vi "ITC panel controller.vi"(6 "itc box state":T1={"ITC503 Address"="GPIB0::15::INSTR", "ITC temperature"=0.0, "ITC set temperature"=300.0, "heater"=300.0, "gas flow"=1.6, "P"=0.0, "D"=10.0, "I"=0.1, "ITC state"="X0A1C2S01H1L0\r", "nonzero temperature"=0.0, "Magn Field (T)"=0.0}, 7 "action":T4(ring), 8 "ITC panel IN":refnum<vi>, 11 "ITC panel IN":T5={"Locked"=FALSE, "Unlocked"=FALSE, "Remote"=FALSE, "Local"=FALSE, "in sweep"=FALSE, "start/stop sweep"=FALSE, "Sweep indicator"="X0A1C2S01H1L0\r", "heater MANUAL"=FALSE, "heater AUTO"=FALSE, "ITC state"="X0A1C2S01H1L0\r", "gas MANUAL"=FALSE, "gas AUTO"=FALSE, "heater"=13.5, "gas flow %"=0.0} {"gas flow %" format="%.3g"; "heater" format="%.3g"}) -> (3 "ITC panel OUT":T5={"Locked"=FALSE, "Unlocked"=FALSE, "Remote"=FALSE, "Local"=FALSE, "in sweep"=FALSE, "start/stop sweep"=FALSE, "Sweep indicator"="X0A1C2S01H1L0\r", "heater MANUAL"=FALSE, "heater AUTO"=FALSE, "ITC state"="X0A1C2S01H1L0\r", "gas MANUAL"=FALSE, "gas AUTO"=FALSE, "heater"=13.5, "gas flow %"=0.0} {"gas flow %" format="%.3g"; "heater" format="%.3g"})   [LabVIEW 2014]
uses:
  ITC Panel.ctl
  state.ctl
  Sample_Temperature_Source_Control.ctl
  itc 503 box state.ctl
  <vilib>/regexp/Match Regular Expression.xnode
panel:
  in  "temperature boxes":T2={"LTC21 Address"="GPIB0::15::INSTR", "ITC503 Address"="GPIB0::23::INSTR", "ITC temperature"=480.0, "ITC set temperature"=480.0, "LTC temperature"=0.0, "heater"=13.5, "gas flow"=0.0, "P"=10.0, "D"=1.0, "I"=3.0, "ITC state"="X0A1C2S01H1L0\r", "nonzero temperature"=0.0, "Magn Field (T)"=0.0, "LakeShore340"="", "LS340 Adress"=0, "Sample Temperature Source"=enum."read T <- LakeShore 340", "Neocera sensor"=1}
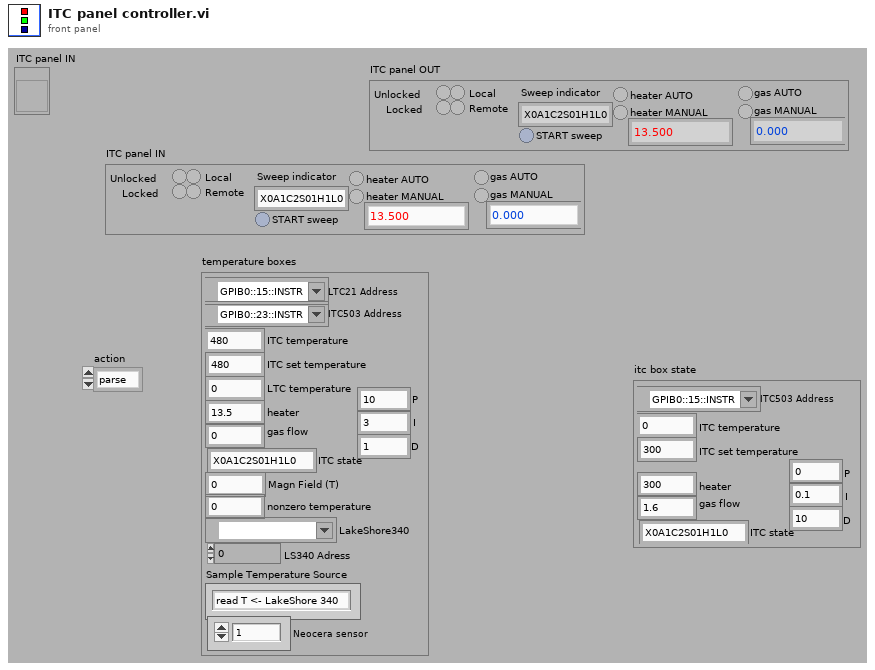
[diagram p1: front panel]
types:
  T1 = typedef "itc 503 box state.ctl" = cluster{"ITC503 Address":refnum<visa-resource-name>, "ITC temperature":dbl, "ITC set temperature":dbl, "heater":dbl, "gas flow":dbl, "P":dbl, "D":dbl, "I":dbl, "ITC state":string, "nonzero temperature":dbl, "Magn Field (T)":dbl}
  T2 = typedef "state.ctl" = cluster{"LTC21 Address":refnum<visa-resource-name>, "ITC503 Address":refnum<visa-resource-name>, "ITC temperature":dbl, "ITC set temperature":dbl, "LTC temperature":dbl, "heater":dbl, "gas flow":dbl, "P":dbl, "D":dbl, "I":dbl, "ITC state":string, "nonzero temperature":dbl, "Magn Field (T)":dbl, "LakeShore340":refnum<visa-resource-name>, "LS340 Adress":i16, "Sample Temperature Source":T3, "Neocera sensor":i32}
  T3 = typedef "Sample_Temperature_Source_Control.ctl" = enum16{"read T <- LakeShore 340", "read T <- Neocera"}
  T4 = enum16{"parse", "start sweep", "stop sweep", "heater auto", "heater manual", "set heater"}
  T5 = typedef "ITC Panel.ctl" = cluster{"Locked":bool, "Unlocked":bool, "Remote":bool, "Local":bool, "in sweep":bool, "start/stop sweep":bool, "Sweep indicator":string, "heater MANUAL":bool, "heater AUTO":bool, "ITC state":string, "gas MANUAL":bool, "gas AUTO":bool, "heater":dbl, "gas flow %":dbl}
  T6 = cluster{"Locked":bool, "Unlocked":bool, "Remote":bool, "Local":bool, "in sweep":bool, "start/stop sweep":bool, "Sweep indicator":string, "heater MANUAL":bool, "heater AUTO":bool, "ITC state":string, "gas MANUAL":bool, "gas AUTO":bool, "heater":dbl, "gas flow %":dbl}
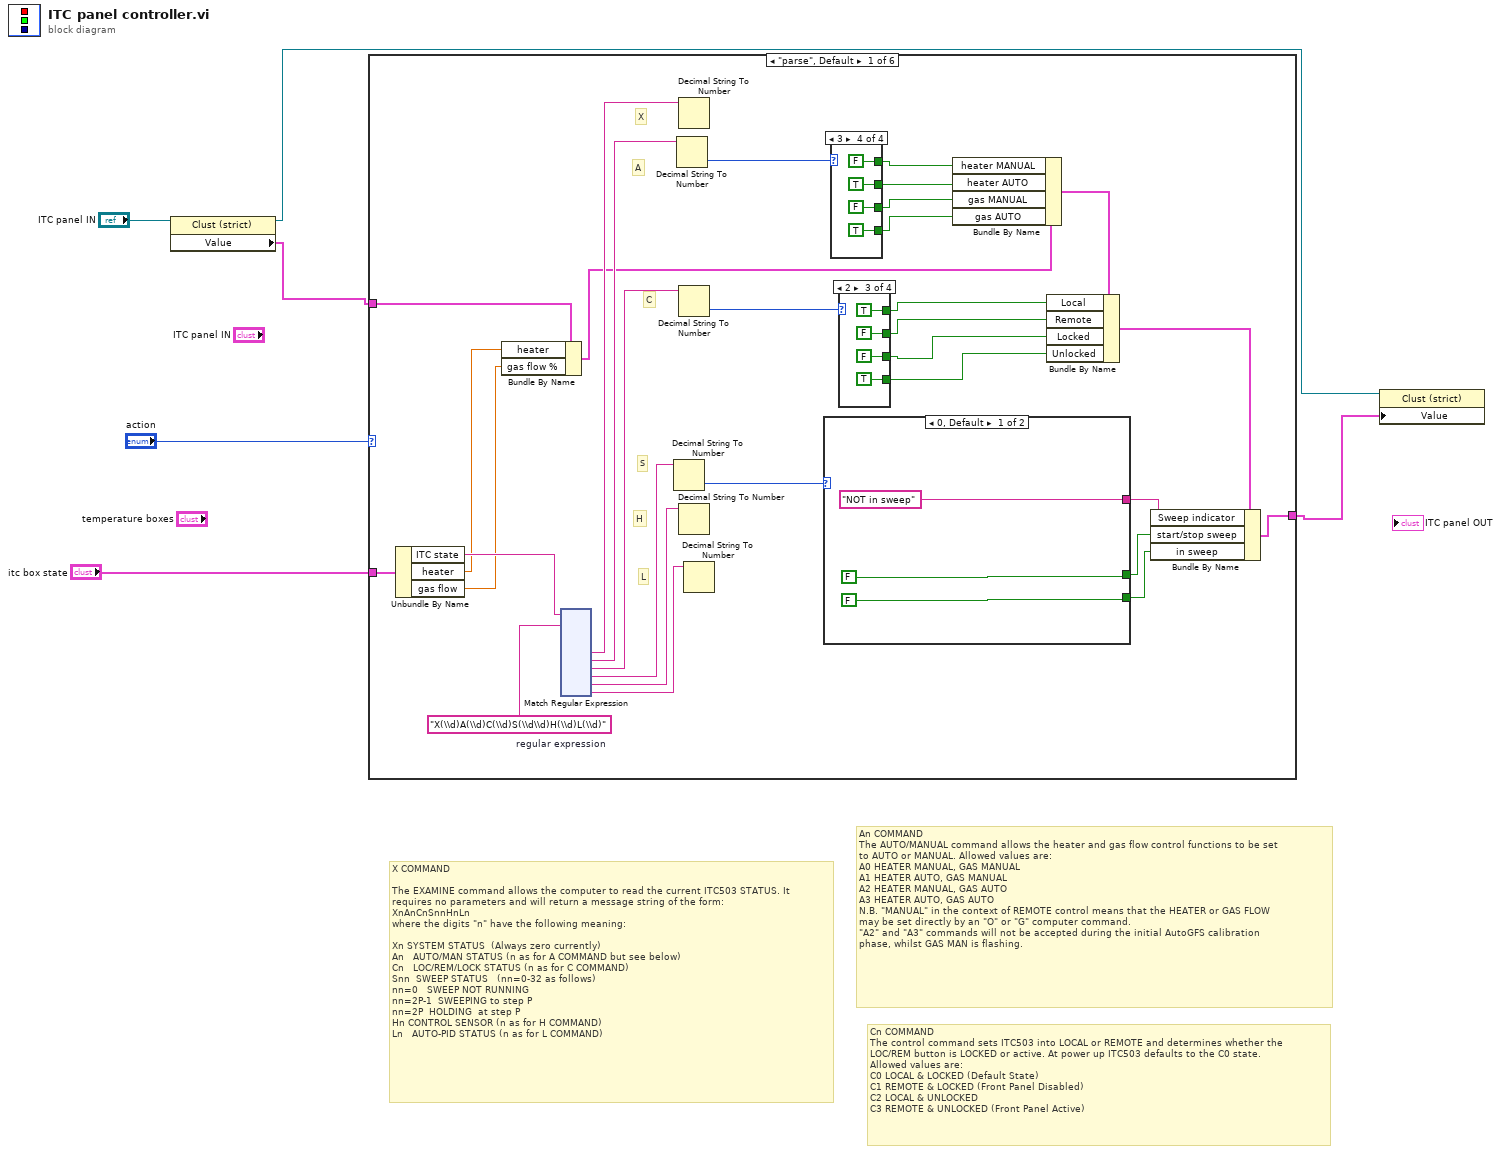
[diagram p0: block diagram]
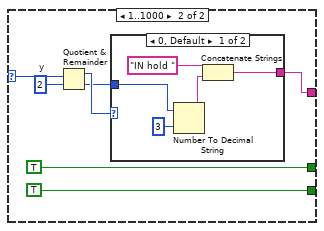
[diagram p2: hidden frame]
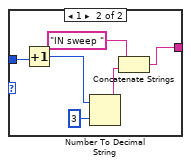
[diagram p3: hidden frame]
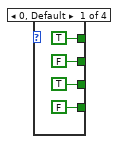
[diagram p4: hidden frame]
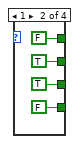
[diagram p5: hidden frame]
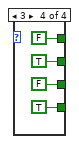
[diagram p6: hidden frame]
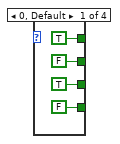
[diagram p7: hidden frame]
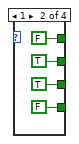
[diagram p8: hidden frame]
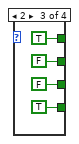
[diagram p9: hidden frame]
diagram:
  # "Cn COMMAND\nThe control command sets ITC503 into LOCAL or REMOTE and determines whether the\nLOC/REM button is LOCKED or active. At power up ITC503 defaults to the C0 state.\nAllowed values are:\nC0 LOCAL & LOCKED (Default State)\nC1 REMOTE & LOCKED (Front Panel Disabled)\nC2 LOCAL & UNLOCKED\nC3 REMOTE & UNLOCKED (Front Panel Active)"
  # "An COMMAND\nThe AUTO/MANUAL command allows the heater and gas flow control functions to be set\nto AUTO or MANUAL. Allowed values are:\nA0 HEATER MANUAL, GAS MANUAL\nA1 HEATER AUTO, GAS MANUAL\nA2 HEATER MANUAL, GAS AUTO\nA3 HEATER AUTO, GAS AUTO\nN.B. \"MANUAL\" in the context of REMOTE control means that the HEATER or GAS FLOW\nmay be set directly by an \"O\" or \"G\" computer command.\n\"A2\" and \"A3\" commands will not be accepted during the initial AutoGFS calibration\nphase, whilst GAS MAN is flashing."
  # "X COMMAND\n\nThe EXAMINE command allows the computer to read the current ITC503 STATUS. It\nrequires no parameters and will return a message string of the form:\nXnAnCnSnnHnLn\nwhere the digits \"n\" have the following meaning:\n\nXn SYSTEM STATUS  (Always zero currently)\nAn   AUTO/MAN STATUS (n as for A COMMAND but see below)\nCn   LOC/REM/LOCK STATUS (n as for C COMMAND)\nSnn  SWEEP STATUS   (nn=0-32 as follows)\nnn=0   SWEEP NOT RUNNING\nnn=2P-1  SWEEPING to step P\nnn=2P  HOLDING  at step P\nHn CONTROL SENSOR (n as for H COMMAND)\nLn   AUTO-PID STATUS (n as for L COMMAND)"
  n1 = property class="Clust (strict)"(reference="ITC panel IN") -> (reference out=w3:refnum<vi>, "Value"=w4:T6)  [unwired: 1 in, 1 out]
  n2 = case shown="\"parse\", Default" "action" {
    tunnel: "itc box state" -> [w16 _ _ _ _ _]
    tunnel: [w17 w208 w209 w210 w211 w212] -> w2
    tunnel: w4 -> [w12 w208 w209 w210 w211 w212]
    frame "parse", Default {
      w36 = "X(\\d)A(\\d)C(\\d)S(\\d\\d)H(\\d)L(\\d)"  # regular expression
      # "L"
      # "H"
      # "S"
      # "C"
      # "A"
      # "X"
      n3 = Unbundle By Name(w16) -> ("ITC state"=w15:string, "heater"=w11:dbl, "gas flow"=w10:dbl)
      n4 = Bundle By Name(cluster=w12, "heater"=w11, "gas flow %"=w10) -> (w9:T6)
      n5 = xnode "Match Regular Expression"("input string"=w15, "regular expression"=w36) -> ("submatch 1"=w35:string, "submatch 2"=w34:string, "submatch 3"=w33:string, "submatch 4"=w32:string, "submatch 5"=w31:string, "submatch 6"=w30:string)  [unwired: 4 in, 5 out]
      n6 = Decimal String To Number(string=w32) -> (number=w20:i32)  [unwired: 2 in, 1 out]
      n7 = Decimal String To Number(string=w34) -> (number=w29:i32)  [unwired: 2 in, 1 out]
      n8 = Decimal String To Number(string=w35) -> ()  [unwired: 2 in, 2 out]
      n9 = Decimal String To Number(string=w33) -> (number=w25:i32)  [unwired: 2 in, 1 out]
      n10 = Decimal String To Number(string=w31) -> ()  [unwired: 2 in, 2 out]
      n11 = Decimal String To Number(string=w30) -> ()  [unwired: 2 in, 2 out]
      n12 = case shown="0, Default" w20 {
        selector: w20 -> [_ w44]
        tunnel: [FALSE TRUE] -> w8
        tunnel: [FALSE TRUE] -> w7
        tunnel: ["NOT in sweep" ("regular expression") w41] -> w18
        frame 0, Default {
        }
        frame 1..1000 {
          w43 = 2  # y
          n13 = Quotient & Remainder(x=w44, y=w43) -> (x-y*floor(x/y)=w42:i32, floor(x/y)=w40:i32)
          n14 = case shown="0, Default" w42 {
            tunnel: [w50 w52] -> w41
            tunnel: w40 -> [w48 w57]
            frame 0, Default {
              n15 = Number To Decimal String(number=w48, width (-)=i16 3) -> (decimal integer string=w49:string)
              n16 = Concatenate Strings("IN hold " ("regular expression"), w49) -> (w50:string)
            }
            frame 1 {
              n17 = Increment(x=w57) -> (x+1=w53:i32)
              n18 = Number To Decimal String(number=w53, width (-)=i16 3) -> (decimal integer string=w55:string)
              n19 = Concatenate Strings("IN sweep " ("regular expression"), w55) -> (w52:string)
            }
          }
        }
      }
      n20 = case shown="3" w29 {
        tunnel: [TRUE FALSE TRUE FALSE] -> w28
        tunnel: [FALSE TRUE FALSE TRUE] -> w27
        tunnel: [TRUE TRUE FALSE FALSE] -> w14
        tunnel: [FALSE FALSE TRUE TRUE] -> w13
        frame 0, Default {
        }
        frame 1 {
        }
        frame 2 {
        }
        frame 3 {
        }
      }
      n21 = case shown="2" w25 {
        tunnel: [TRUE FALSE TRUE FALSE] -> w24
        tunnel: [FALSE TRUE FALSE TRUE] -> w23
        tunnel: [TRUE TRUE FALSE FALSE] -> w22
        tunnel: [FALSE FALSE TRUE TRUE] -> w21
        frame 0, Default {
        }
        frame 1 {
        }
        frame 2 {
        }
        frame 3 {
        }
      }
      n22 = Bundle By Name(cluster=w9, "heater MANUAL"=w28, "heater AUTO"=w27, "gas MANUAL"=w14, "gas AUTO"=w13) -> (w26:T6)
      n23 = Bundle By Name(cluster=w26, "Local"=w24, "Remote"=w23, "Locked"=w22, "Unlocked"=w21) -> (w19:T6)
      n24 = Bundle By Name(cluster=w19, "Sweep indicator"=w18, "start/stop sweep"=w8, "in sweep"=w7) -> (w17:T6)
    }
    frame "start sweep" {
    }
    frame "stop sweep" {
    }
    frame "heater auto" {
    }
    frame "heater manual" {
    }
    frame "set heater" {
    }
  }
  n25 = property class="Clust (strict)"(reference=w3, "Value"=w2) -> ()  [unwired: 1 in, 2 out]
